vi "Configuration File Get VeriStand Application Path.vi"(8 "error in (no error)":errorcluster) -> (0 "error out":errorcluster, 2 "Found?":bool, 3 "VeriStand Application Path":path)   [LabVIEW 2015, in "ni-veristand-steps-runtime-lib.lvlib"]
uses:
  ni-veristand-steps-runtime-lib.lvlib
  <vilib>/Utility/config.llb/Read Key (String).vi
  <vilib>/Utility/config.llb/NI_LVConfig.lvlib
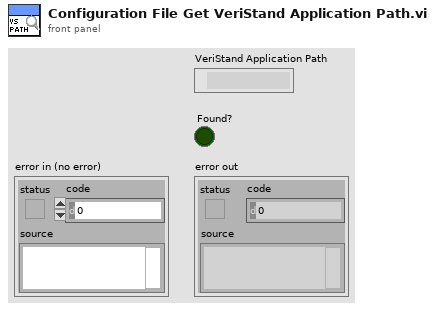
[diagram p1: front panel]
types:
  T1 = typedef "NI_LVConfig.lvlib/Config Data RefNum.ctl" = refnum<k1>
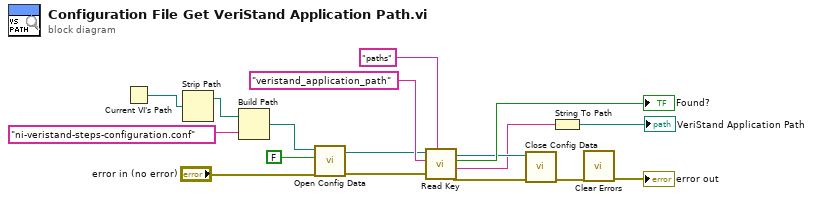
[diagram p0: block diagram]
diagram:
  n1 = Current VI's Path() -> (path=w15:path)
  n2 = Strip Path(path=w15) -> (stripped path=w16:path)  [unwired: 1 out]
  n3 = Build Path(base path=w16, name or relative path="ni-veristand-steps-configuration.conf") -> (appended path=w7:path)
  n4 = call <vilib>:"Open Config Data.vi"("error in (no error)"="error in (no error)", "create file if necessary (T)"=FALSE, "configuration file path"=w7) -> ("error out"=w10:errorcluster, "refnum"=w9:T1)  [unwired: 6 in, 1 out]
  n5 = call-poly <vilib>:"Read Key.vi"("section"="paths", "error in (no error)"=w10, "key"="veristand_application_path", "refnum"=w9) -> ("error out"=w14:errorcluster, "value"=w2:string, "found?"=→"Found?":bool, "refnum out"=w13:T1)  [unwired: 4 in]
  n6 = call <vilib>:"Close Config Data.vi"("error in (no error)"=w14, "refnum"=w13) -> ("error out"=w4:errorcluster)  [unwired: 8 in, 1 out]
  n7 = String To Path(string=w2) -> (path=→"VeriStand Application Path":path)
  n8 = call <vilib>:"Clear Errors.vi"("error in (no error)"=w4) -> ("error out"=→"error out":errorcluster)  [unwired: 5 in, 1 out]
